vi "write_sine.vi"() -> ()   [LabVIEW 2020]
panel:
  in  "Phase (deg)":dbl
  out "output control error":errorcluster
  out "configure error out":errorcluster
  in  "Output 2":bool
  in  "Output 1":bool
  in  "Channel Selection":u16(ring) items=["Channel 1", "Channel 2"]
  in  "Frequency (Hz)":dbl=1000.0
  in  "DC Offset (0.00 V)":dbl
  in  "Amplitude (1)":dbl=1.0
  in  "?":bool
  in  "?":bool
  in  "VISA resource name":refnum<visa-resource-name>
  # "Rigol Technologies DG4/DG1Z General"
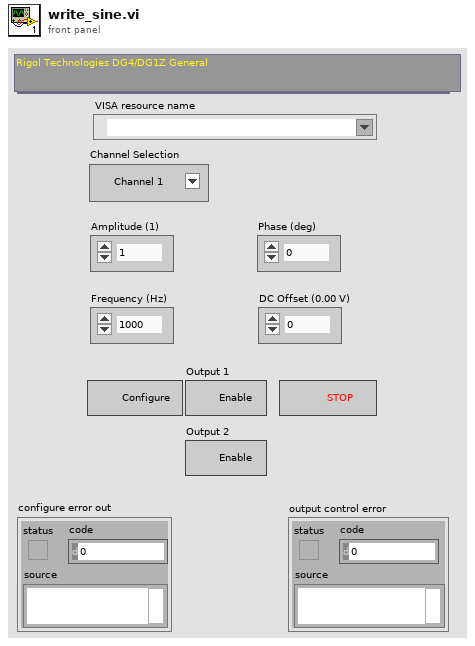
[diagram p1: front panel]
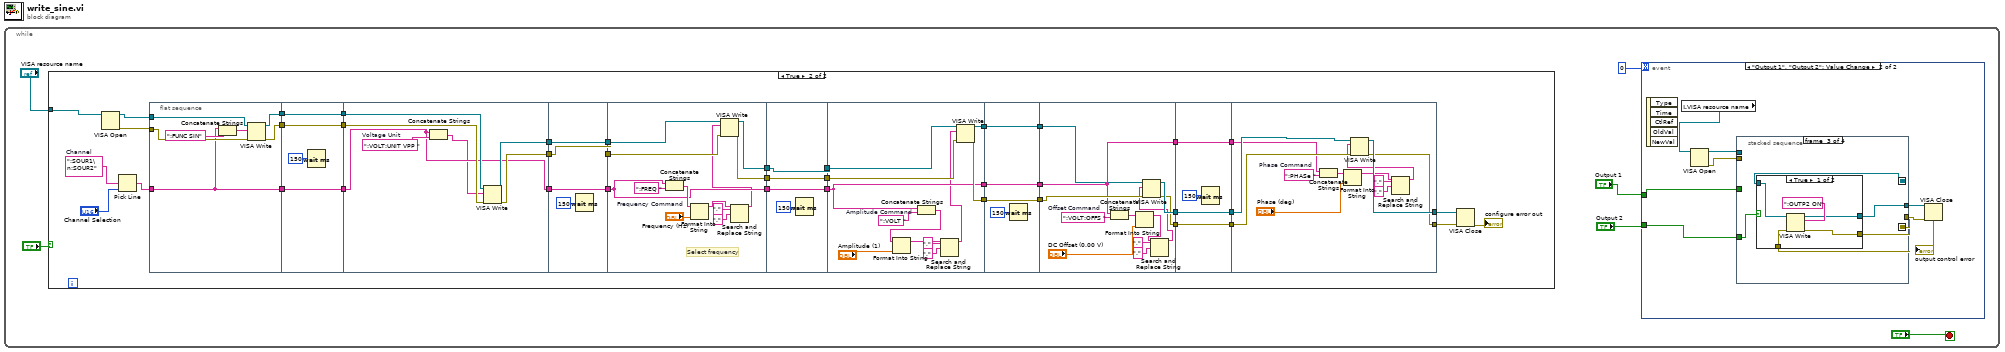
[diagram p0: block diagram]
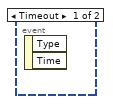
[diagram p2: hidden frame]
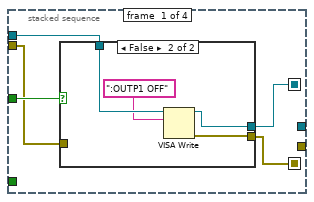
[diagram p3: hidden frame]
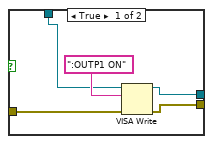
[diagram p4: hidden frame]
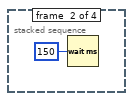
[diagram p5: hidden frame]
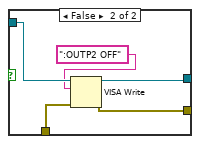
[diagram p6: hidden frame]
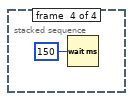
[diagram p7: hidden frame]
diagram:
  n1 = while {
    stop <- "?" stop-if-true
    n2 = case shown="True" "?" {
      tunnel: "VISA resource name" -> [_ w83]
      frame False {
      }
      frame True {
        w76 = ":SOUR1\n:SOUR2"  # Channel
        n3 = VISA Open(VISA resource name=w83) -> (VISA resource name=w82:refnum<visa-resource-name>, error out=w84:errorcluster)  [unwired: 4 in]
        n4 = Pick Line(multi-line string=w76, line index="Channel Selection") -> (output string=w78:string)  [unwired: 1 in]
        n5 = flat-sequence {
          tunnel: w82 -> [w91]
          tunnel: w84 -> [w90]
          tunnel: w78 -> [w86]
          tunnel: [w86] -> w75
          tunnel: [w87] -> w74
          tunnel: [w88] -> w73
          tunnel: w75 -> [w94]
          tunnel: [w94] -> w72
          tunnel: w74 -> [w93]
          tunnel: [w93] -> w71
          tunnel: w73 -> [w92]
          tunnel: [w92] -> w70
          tunnel: w72 -> [w97]
          tunnel: [w97] -> w69
          tunnel: w71 -> [w101]
          tunnel: w70 -> [w100]
          tunnel: [w99] -> w68
          tunnel: [w98] -> w67
          tunnel: w69 -> [w105]
          tunnel: [w105] -> w66
          tunnel: w68 -> [w104]
          tunnel: [w104] -> w65
          tunnel: w67 -> [w103]
          tunnel: [w103] -> w64
          tunnel: w66 -> [w111]
          tunnel: [w111] -> w63
          tunnel: w65 -> [w115]
          tunnel: w64 -> [w114]
          tunnel: [w113] -> w62
          tunnel: [w112] -> w61
          tunnel: w63 -> [w121]
          tunnel: [w121] -> w60
          tunnel: w62 -> [w120]
          tunnel: [w120] -> w59
          tunnel: w61 -> [w119]
          tunnel: [w119] -> w58
          tunnel: w60 -> [w127]
          tunnel: [w127] -> w57
          tunnel: w59 -> [w131]
          tunnel: w58 -> [w130]
          tunnel: [w129] -> w56
          tunnel: [w128] -> w55
          tunnel: w57 -> [w137]
          tunnel: [w137] -> w54
          tunnel: w56 -> [w136]
          tunnel: [w136] -> w53
          tunnel: w55 -> [w135]
          tunnel: [w135] -> w52
          tunnel: [w145] -> w51
          tunnel: [w144] -> w50
          tunnel: w54 -> [w143]
          tunnel: w53 -> [w147]
          tunnel: w52 -> [w146]
          tunnel: [w143] -> w46
          tunnel: w51 -> [w153]
          tunnel: w50 -> [w152]
          tunnel: [w153] -> w49
          tunnel: [w152] -> w48
          tunnel: [w151] -> w47
          tunnel: w46 -> [w151]
          tunnel: [w160] -> w80
          tunnel: [w162] -> w81
          tunnel: w49 -> [w163]
          tunnel: w48 -> [w161]
          tunnel: w47 -> [w156]
          frame #0 {
            n6 = Concatenate Strings(w86, ":FUNC SIN" ("string (\"\")")) -> (w85:string)
            n7 = VISA Write(VISA resource name=w91, write buffer=w85, error in (no error)=w90) -> (VISA resource name out=w87:refnum<visa-resource-name>, error out=w88:errorcluster)  [unwired: 1 out]
          }
          frame #1 {
            n8 = Wait (ms)(milliseconds to wait=u32 150) -> ()  [unwired: 1 out]
          }
          frame #2 {
            w102 = ":VOLT:UNIT VPP "  # Voltage Unit
            n9 = Concatenate Strings(w97, w102) -> (w96:string)
            n10 = VISA Write(VISA resource name=w101, write buffer=w96, error in (no error)=w100) -> (VISA resource name out=w99:refnum<visa-resource-name>, error out=w98:errorcluster)  [unwired: 1 out]
          }
          frame #3 {
            n11 = Wait (ms)(milliseconds to wait=u32 150) -> ()  [unwired: 1 out]
          }
          frame #4 {
            w117 = ":FREQ "  # Frequency Command
            # "Select frequency"
            n12 = Concatenate Strings(w111, w117) -> (w116:string)
            n13 = Format Into String(initial string=w116, "Frequency (Hz)") -> (resulting string=w108:string)  [unwired: 2 in, 1 out]
            n14 = Search and Replace String(input string=w108, search string=",", replace string="." ("replace string (\"\")")) -> (result string=w107:string)  [unwired: 5 in, 3 out]
            n15 = VISA Write(VISA resource name=w115, write buffer=w107, error in (no error)=w114) -> (VISA resource name out=w113:refnum<visa-resource-name>, error out=w112:errorcluster)  [unwired: 1 out]
          }
          frame #5 {
            n16 = Wait (ms)(milliseconds to wait=u32 150) -> ()  [unwired: 1 out]
          }
          frame #6 {
            w133 = ":VOLT "  # Amplitude Command
            n17 = Concatenate Strings(w127, w133) -> (w132:string)
            n18 = Format Into String(initial string=w132, "Amplitude (1)") -> (resulting string=w126:string)  [unwired: 2 in, 1 out]
            n19 = Search and Replace String(input string=w126, search string=",", replace string="." ("replace string (\"\")")) -> (result string=w123:string)  [unwired: 5 in, 3 out]
            n20 = VISA Write(VISA resource name=w131, write buffer=w123, error in (no error)=w130) -> (VISA resource name out=w129:refnum<visa-resource-name>, error out=w128:errorcluster)  [unwired: 1 out]
          }
          frame #7 {
            n21 = Wait (ms)(milliseconds to wait=u32 150) -> ()  [unwired: 1 out]
          }
          frame #8 {
            w149 = ":VOLT:OFFS "  # Offset Command
            n22 = Concatenate Strings(w143, w149) -> (w148:string)
            n23 = Format Into String(initial string=w148, "DC Offset (0.00 V)") -> (resulting string=w141:string)  [unwired: 2 in, 1 out]
            n24 = Search and Replace String(input string=w141, search string=",", replace string="." ("replace string (\"\")")) -> (result string=w139:string)  [unwired: 5 in, 3 out]
            n25 = VISA Write(VISA resource name=w147, write buffer=w139, error in (no error)=w146) -> (VISA resource name out=w145:refnum<visa-resource-name>, error out=w144:errorcluster)  [unwired: 1 out]
          }
          frame #9 {
            n26 = Wait (ms)(milliseconds to wait=u32 150) -> ()  [unwired: 1 out]
          }
          frame #10 {
            w165 = ":PHASe "  # Phase Command
            n27 = Concatenate Strings(w156, w165) -> (w164:string)
            n28 = Format Into String(initial string=w164, "Phase (deg)") -> (resulting string=w157:string)  [unwired: 2 in, 1 out]
            n29 = Search and Replace String(input string=w157, search string=",", replace string="." ("replace string (\"\")")) -> (result string=w155:string)  [unwired: 5 in, 3 out]
            n30 = VISA Write(VISA resource name=w163, write buffer=w155, error in (no error)=w161) -> (VISA resource name out=w162:refnum<visa-resource-name>, error out=w160:errorcluster)  [unwired: 1 out]
          }
        }
        n31 = VISA Close(VISA resource name=w81, error in (no error)=w80) -> (error out=→"configure error out":errorcluster)
      }
    }
    n32 = event shown="[1] \"Output 1\", \"Output 2\": Value Change" {
      selector: _ -> [_ _]
      dyn-events: _ -> [_ _]
      timeout: u32 0 ("Time") -> [_ _]
      tunnel: "Output 2" -> [_ w14]
      tunnel: "Output 1" -> [_ w13]
      event Timeout {
        n33 = event-data() -> ()  [unwired: 1 in, 2 out]
      }
      event "Output 1", "Output 2": Value Change {
        n34 = event-data() -> ()  [unwired: 1 in, 5 out]
        n35 = local read "VISA resource name"() -> (w12:refnum<visa-resource-name>)
        n36 = VISA Open(VISA resource name=w12) -> (VISA resource name=w11:refnum<visa-resource-name>, error out=w10:errorcluster)  [unwired: 4 in]
        n37 = stacked-sequence {
          seq-local: [w17 _ _ _] -> [_ _ w33 _]
          seq-local: [w15 _ _ _] -> [_ _ w31 _]
          tunnel: w11 -> [w19 _ _ _]
          tunnel: w14 -> [_ _ w34 _]
          tunnel: w13 -> [w18 _ _ _]
          tunnel: [_ _ w32 _] -> w9
          tunnel: w10 -> [w16 _ _ _]
          tunnel: [_ _ w30 _] -> w8
          frame #0 {
            n38 = case shown="False" w18 {
              tunnel: w19 -> [w23 w28]
              tunnel: [w22 w26] -> w17
              tunnel: w16 -> [w21 _]
              tunnel: [w20 w25] -> w15
              frame True {
                n39 = VISA Write(VISA resource name=w23, write buffer=":OUTP1 ON", error in (no error)=w21) -> (VISA resource name out=w20:refnum<visa-resource-name>, error out=w22:errorcluster)  [unwired: 1 out]
              }
              frame False {
                n40 = VISA Write(VISA resource name=w28, write buffer=":OUTP1 OFF") -> (VISA resource name out=w25:refnum<visa-resource-name>, error out=w26:errorcluster)  [unwired: 1 in, 1 out]
              }
            }
          }
          frame #1 {
            n41 = Wait (ms)(milliseconds to wait=u32 150) -> ()  [unwired: 1 out]
          }
          frame #2 {
            n42 = case shown="True" w34 {
              tunnel: w31 -> [w38 w44]
              tunnel: [w37 w42] -> w32
              tunnel: w33 -> [w36 w41]
              tunnel: [w35 w40] -> w30
              frame True {
                n43 = VISA Write(VISA resource name=w38, write buffer=":OUTP2 ON", error in (no error)=w36) -> (VISA resource name out=w35:refnum<visa-resource-name>, error out=w37:errorcluster)  [unwired: 1 out]
              }
              frame False {
                n44 = VISA Write(VISA resource name=w44, write buffer=":OUTP2 OFF", error in (no error)=w41) -> (VISA resource name out=w40:refnum<visa-resource-name>, error out=w42:errorcluster)  [unwired: 1 out]
              }
            }
          }
          frame #3 {
            n45 = Wait (ms)(milliseconds to wait=u32 150) -> ()  [unwired: 1 out]
          }
        }
        n46 = VISA Close(VISA resource name=w8, error in (no error)=w9) -> (error out=→"output control error":errorcluster)
      }
    }
  }
